vi "SetFruitRef.vi"(7 "This VI":refnum<vi>, 8 "Error In":errorcluster, 10 "FruitRef":refnum<class "Fruit.lvclass">, 11 "object in":refnum<class "Board Game.lvclass">) -> (0 "Error Out":errorcluster, 3 "object out":refnum<class "Board Game.lvclass">)   [LabVIEW 2021, in "Board Game.lvclass"]
uses:
  Board Game.lvclass
  Fruit_class/Fruit.lvclass
  Board Game.lvclass/Board Game.ctl
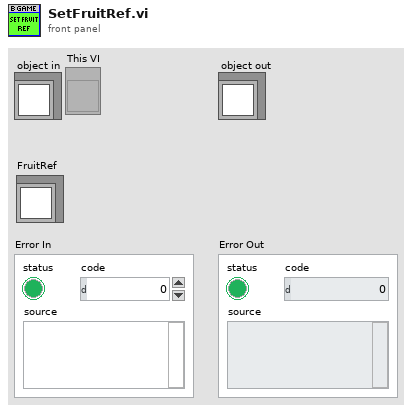
[diagram p1: front panel]
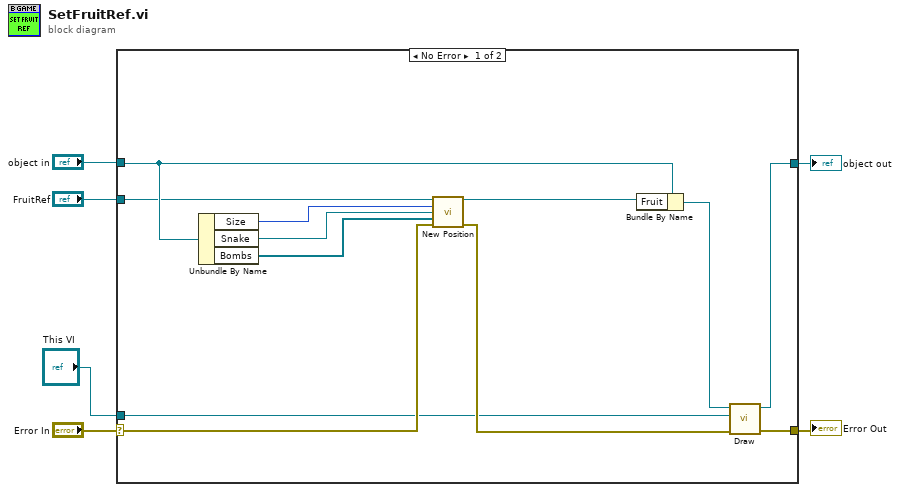
[diagram p0: block diagram]
diagram:
  n1 = case shown="No Error" "Error In" {
    selector: "Error In" -> [w9 w20]
    tunnel: [w18 w20] -> w5
    tunnel: [w15 w19] -> w3
    tunnel: "object in" -> [w17 w19]
    tunnel: "FruitRef" -> [w14 _]
    tunnel: "This VI" -> [w7 _]
    frame No Error {
      n2 = Unbundle By Name(w17) -> ("Size"=w12:u16, "Snake"=w11:refnum<class "Snake.lvclass">, "Bombs"=w8:refnum<class "Bomb.lvclass">[])
      n3 = call "New Position.vi"("Fruit in"=w14, "B Game Size"=w12, "Snake"=w11, "Bomb"=w8, "error in (no error)"=w9) -> ("Fruit out"=w13:refnum<class "Fruit.lvclass">, "error out"=w10:errorcluster)  [unwired: 8 in, 1 out]
      n4 = Bundle By Name(cluster=w17, "Fruit"=w13) -> (w16:refnum<class "Board Game.lvclass">)
      n5 = call "Draw.vi"("error in (no error)"=w10, "This VI"=w7, "Board Game in"=w16) -> ("error out"=w18:errorcluster, "Board Game out"=w15:refnum<class "Board Game.lvclass">)  [unwired: 7 in]
    }
    frame Error {
    }
  }
  "Error Out" <- w5
  "object out" <- w3
